vi "KH_DAQ_TURCK_ScaleAO.vi"(4 "Sollwert":sgl=1000.0, 8 "Bereich":T1=enum."NE43", 9 "Messbereich":T2=enum."+2V ... +10V", 10 "PhysMax":sgl format="%.4f", 11 "PhysMin":sgl format="%.4f") -> (3 "Sollwert Turck":i16)   [LabVIEW 2021]
uses:
  KH_DAQ_TypeDefs_Messbereich.ctl
  KH_DAQ_TypeDefs_Bereich.ctl
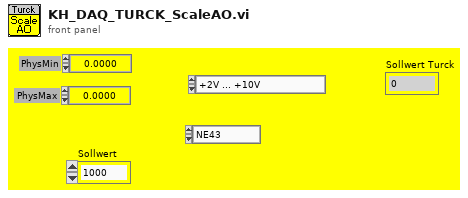
[diagram p1: front panel]
types:
  T1 = typedef "KH_DAQ_TypeDefs_Bereich.ctl" = enum16{"Standard", "extended Range", "NE43", ""}
  T2 = typedef "KH_DAQ_TypeDefs_Messbereich.ctl" = enum16{"-10V ... +10V", "0V ... +10V", "+2V ... +10V", "0V ... +5V", "+1V ... +5V", "-1V ... +1V", "-500mV ... +500mV", "-100mV ... +100mV", "-50mV ... +50mV", "0mA ... +20mA", "+4mA ... +20mA", "-20mA ... +20mA", "0 Ohm ... 100 Ohm", "0 Ohm ... 400 Ohm", "0 Ohm ... 2000 Ohm", "0 Ohm ... 4000 Ohm", "-200°C ... 150°C PT100", "-200°C ... 150°C PT200", "-200°C ... 150°C PT500", "-200°C ... 150°C PT1000", "-60°C ... 150°C Ni100", "-60°C ... 150°C Ni1000", "-200°C ... 850°C PT100", "-200°C ... 850°C PT200", "-200°C ... 850°C PT500", "-200°C ... 850°C PT1000", "-50°C ... 250°C Ni100", "-50°C ... 250° Ni 1000"}
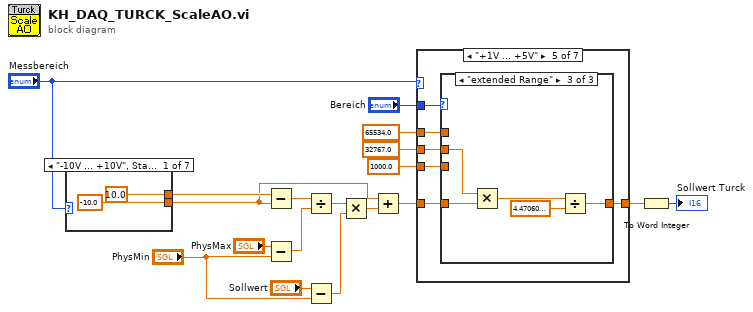
[diagram p0: block diagram]
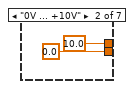
[diagram p2: hidden frame]
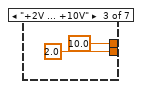
[diagram p3: hidden frame]
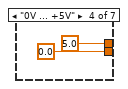
[diagram p4: hidden frame]
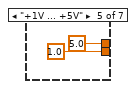
[diagram p5: hidden frame]
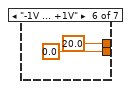
[diagram p6: hidden frame]
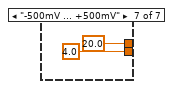
[diagram p7: hidden frame]
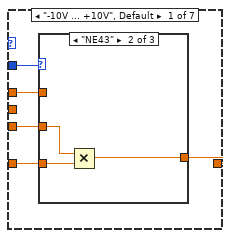
[diagram p8: hidden frame]
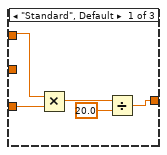
[diagram p9: hidden frame]
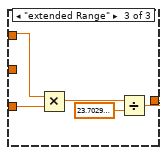
[diagram p10: hidden frame]
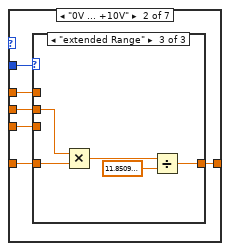
[diagram p11: hidden frame]
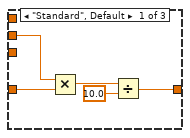
[diagram p12: hidden frame]
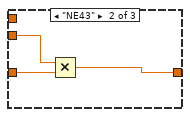
[diagram p13: hidden frame]
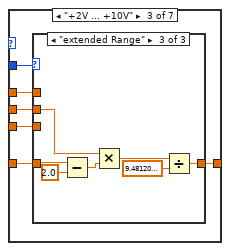
[diagram p14: hidden frame]
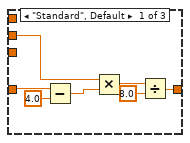
[diagram p15: hidden frame]
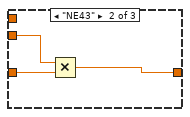
[diagram p16: hidden frame]
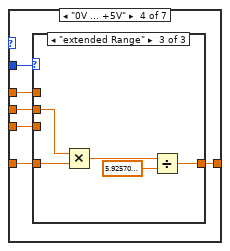
[diagram p17: hidden frame]
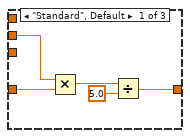
[diagram p18: hidden frame]
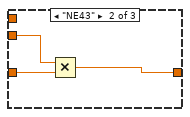
[diagram p19: hidden frame]
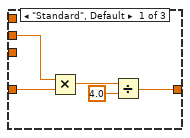
[diagram p20: hidden frame]
diagram:
  n1 = case shown="\"-10V ... +10V\", Standard" "Messbereich" {
    tunnel: [sgl -10.0 ("-10V") sgl 0.0 ("-10V") sgl 2.0 ("-10V") sgl 0.0 ("-10V") sgl 1.0 ("-10V") sgl 0.0 ("-10V") sgl 4.0 ("-10V")] -> w10
    tunnel: [sgl 10.0 ("-10V") sgl 10.0 ("-10V") sgl 10.0 ("-10V") sgl 5.0 ("-10V") sgl 5.0 ("-10V") sgl 20.0 ("-10V") sgl 20.0 ("-10V")] -> w11
    frame "-10V ... +10V", Default {
    }
    frame "0V ... +10V" {
    }
    frame "+2V ... +10V" {
    }
    frame "0V ... +5V" {
    }
    frame "+1V ... +5V" {
    }
    frame "-1V ... +1V" {
    }
    frame "-500mV ... +500mV" {
    }
  }
  n2 = Subtract(x=w11, y=w10) -> (x-y=w9:sgl)
  n3 = Subtract(x="PhysMax", y="PhysMin") -> (x-y=w8:sgl)
  n4 = Divide(x=w9, y=w8) -> (x/y=w7:sgl)
  n5 = Subtract(x="Sollwert", y="PhysMin") -> (x-y=w6:sgl)
  n6 = Multiply(x=w7, y=w6) -> (x*y=w5:sgl)
  n7 = Add(x=w10, y=w5) -> (x+y=w1:sgl)
  n8 = case shown="\"+1V ... +5V\"" "Messbereich" {
    tunnel: "Bereich" -> [w37 w56 w75 w98 w117 w136 w155]
    tunnel: sgl 65534.0 ("Sollwert 2") -> [w36 w55 w74 w97 w116 w135 w154]
    tunnel: w1 -> [w35 w54 w73 w96 w115 w134 w153]
    tunnel: [w33 w51 w70 w93 w112 w131 w150] -> w17
    tunnel: sgl 32767.0 ("Sollwert 2") -> [_ w52 w71 w94 w113 w132 w151]
    tunnel: sgl 1000.0 ("Sollwert 2") -> [w34 w53 w72 w95 w114 w133 w152]
    frame "-10V ... +10V", Default {
      n9 = case shown="\"NE43\"" w37 {
        tunnel: w36 -> [w41 _ w49]
        tunnel: w35 -> [w42 w45 w50]
        tunnel: [w38 w44 w46] -> w33
        tunnel: w34 -> [_ w43 _]
        frame "Standard", Default {
          n10 = Multiply(x=w41, y=w42) -> (x*y=w39:sgl)
          n11 = Divide(x=w39, y=sgl 20.0 ("Sollwert 2")) -> (x/y=w38:sgl)
        }
        frame "NE43" {
          n12 = Multiply(x=w43, y=w45) -> (x*y=w44:sgl)
        }
        frame "extended Range" {
          n13 = Multiply(x=w49, y=w50) -> (x*y=w47:sgl)
          n14 = Divide(x=w47, y=sgl 23.703 ("Sollwert 2")) -> (x/y=w46:sgl)
        }
      }
    }
    frame "0V ... +10V" {
      n15 = case shown="\"extended Range\"" w56 {
        tunnel: w55 -> [_ _ _]
        tunnel: w54 -> [w61 w63 w69]
        tunnel: [w57 w64 w65] -> w51
        tunnel: w53 -> [_ w62 _]
        tunnel: w52 -> [w60 _ w68]
        frame "Standard", Default {
          n16 = Multiply(x=w60, y=w61) -> (x*y=w58:sgl)
          n17 = Divide(x=w58, y=sgl 10.0 ("Sollwert 2")) -> (x/y=w57:sgl)
        }
        frame "NE43" {
          n18 = Multiply(x=w62, y=w63) -> (x*y=w64:sgl)
        }
        frame "extended Range" {
          n19 = Multiply(x=w68, y=w69) -> (x*y=w66:sgl)
          n20 = Divide(x=w66, y=sgl 11.851 ("Sollwert 2")) -> (x/y=w65:sgl)
        }
      }
    }
    frame "+2V ... +10V" {
      n21 = case shown="\"extended Range\"" w75 {
        tunnel: w74 -> [_ _ _]
        tunnel: w73 -> [w78 w84 w86]
        tunnel: [w79 w85 w89] -> w70
        tunnel: w72 -> [_ w83 _]
        tunnel: w71 -> [w82 _ w92]
        frame "Standard", Default {
          n22 = Subtract(x=w78, y=sgl 4.0) -> (x-y=w77:sgl)
          n23 = Multiply(x=w82, y=w77) -> (x*y=w80:sgl)
          n24 = Divide(x=w80, y=sgl 8.0 ("Sollwert 2")) -> (x/y=w79:sgl)
        }
        frame "NE43" {
          n25 = Multiply(x=w83, y=w84) -> (x*y=w85:sgl)
        }
        frame "extended Range" {
          n26 = Subtract(x=w86, y=sgl 2.0) -> (x-y=w87:sgl)
          n27 = Multiply(x=w92, y=w87) -> (x*y=w90:sgl)
          n28 = Divide(x=w90, y=sgl 9.4812 ("Sollwert 2")) -> (x/y=w89:sgl)
        }
      }
    }
    frame "0V ... +5V" {
      n29 = case shown="\"extended Range\"" w98 {
        tunnel: w97 -> [_ _ _]
        tunnel: w96 -> [w103 w105 w111]
        tunnel: [w99 w106 w107] -> w93
        tunnel: w95 -> [_ w104 _]
        tunnel: w94 -> [w102 _ w110]
        frame "Standard", Default {
          n30 = Multiply(x=w102, y=w103) -> (x*y=w100:sgl)
          n31 = Divide(x=w100, y=sgl 5.0 ("Sollwert 2")) -> (x/y=w99:sgl)
        }
        frame "NE43" {
          n32 = Multiply(x=w104, y=w105) -> (x*y=w106:sgl)
        }
        frame "extended Range" {
          n33 = Multiply(x=w110, y=w111) -> (x*y=w108:sgl)
          n34 = Divide(x=w108, y=sgl 5.9257 ("Sollwert 2")) -> (x/y=w107:sgl)
        }
      }
    }
    frame "+1V ... +5V" {
      n35 = case shown="\"extended Range\"" w117 {
        tunnel: w116 -> [_ _ _]
        tunnel: w115 -> [w122 w124 w130]
        tunnel: [w118 w125 w126] -> w112
        tunnel: w114 -> [_ w123 _]
        tunnel: w113 -> [w121 _ w129]
        frame "Standard", Default {
          n36 = Multiply(x=w121, y=w122) -> (x*y=w119:sgl)
          n37 = Divide(x=w119, y=sgl 4.0 ("Sollwert 2")) -> (x/y=w118:sgl)
        }
        frame "NE43" {
          n38 = Multiply(x=w123, y=w124) -> (x*y=w125:sgl)
        }
        frame "extended Range" {
          n39 = Multiply(x=w129, y=w130) -> (x*y=w127:sgl)
          n40 = Divide(x=w127, y=sgl 4.4706 ("Sollwert 2")) -> (x/y=w126:sgl)
        }
      }
    }
    frame "-1V ... +1V" {
      n41 = case shown="\"extended Range\"" w136 {
        tunnel: w135 -> [_ _ _]
        tunnel: w134 -> [w141 w143 w149]
        tunnel: [w137 w144 w145] -> w131
        tunnel: w133 -> [_ w142 _]
        tunnel: w132 -> [w140 _ w148]
        frame "Standard", Default {
          n42 = Multiply(x=w140, y=w141) -> (x*y=w138:sgl)
          n43 = Divide(x=w138, y=sgl 20.0 ("Sollwert 2")) -> (x/y=w137:sgl)
        }
        frame "NE43" {
          n44 = Multiply(x=w142, y=w143) -> (x*y=w144:sgl)
        }
        frame "extended Range" {
          n45 = Multiply(x=w148, y=w149) -> (x*y=w146:sgl)
          n46 = Divide(x=w146, y=sgl 23.703 ("Sollwert 2")) -> (x/y=w145:sgl)
        }
      }
    }
    frame "-500mV ... +500mV" {
      n47 = case shown="\"NE43\"" w155 {
        tunnel: w154 -> [_ _ _]
        tunnel: w153 -> [w157 w164 w168]
        tunnel: [w159 w167 w171] -> w150
        tunnel: w152 -> [_ w166 _]
        tunnel: w151 -> [w162 _ w174]
        frame "Standard", Default {
          n48 = Subtract(x=w157, y=sgl 4.0) -> (x-y=w156:sgl)
          n49 = Multiply(x=w162, y=w156) -> (x*y=w160:sgl)
          n50 = Divide(x=w160, y=sgl 16.0 ("Sollwert 2")) -> (x/y=w159:sgl)
        }
        frame "NE43" {
          n51 = Subtract(x=w164, y=sgl 4.0) -> (x-y=w163:sgl)
          n52 = Multiply(x=w166, y=w163) -> (x*y=w167:sgl)
        }
        frame "extended Range" {
          n53 = Subtract(x=w168, y=sgl 4.0) -> (x-y=w169:sgl)
          n54 = Multiply(x=w174, y=w169) -> (x*y=w172:sgl)
          n55 = Divide(x=w172, y=sgl 18.962 ("Sollwert 2")) -> (x/y=w171:sgl)
        }
      }
    }
  }
  n56 = To Word Integer(number=w17) -> (16bit integer=→"Sollwert Turck":i16)
